vi "formatSubVI.vi"(8 "error in (no error)":errorcluster, 10 "Message":T2, 11 "Current Text":string) -> (0 "error out":errorcluster, 2 "Text Out":string, 9 "Type":T1)   [LabVIEW 2010]
doc: "This VI takes a cluster three pieces of data and formats it into a string.\nIt then concatenates the newly formated string to the end of a a string read in from a text file."
uses:
  Type.ctl
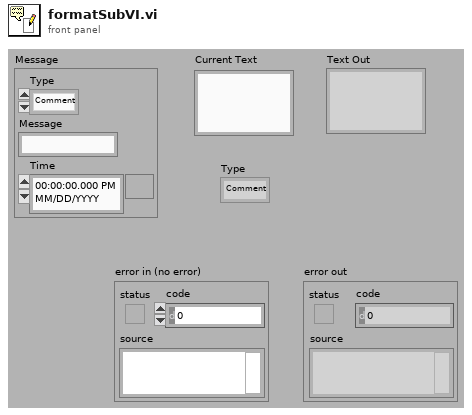
[diagram p1: front panel]
types:
  T1 = typedef "Type.ctl" = enum16{"Comment", "Question", "Concern"}
  T2 = cluster{"Type":T1, "Message":string, "Time":timestamp}
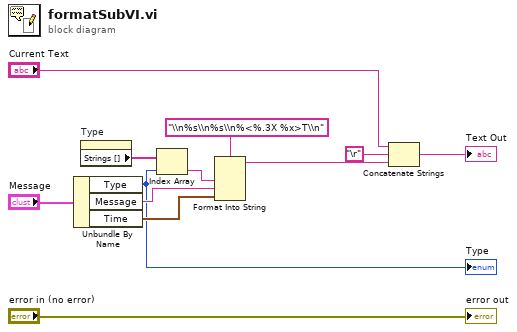
[diagram p0: block diagram]
diagram:
  n1 = Unbundle By Name("Message") -> ("Type"=w1:T1, "Message"=w10:string, "Time"=w11:timestamp)
  "Type" <- w1
  n2 = property on="Type" class="Enum (strict)"() -> ("Strings []"=w7:string[])  [unwired: 2 in, 2 out]
  n3 = Index Array(array=w7, index=w1) -> (element=w8:string)
  n4 = Format Into String(format string="\\n%s\\n%s\\n%<%.3X %x>T\\n", w8, w10, w11) -> (resulting string=w5:string)  [unwired: 2 in, 1 out]
  n5 = Concatenate Strings("Current Text", "\r", w5) -> (→"Text Out":string)
  "error out" <- "error in (no error)"
